vi "Begin.vi"(8 "error in":errorcluster) -> (0 "error out":errorcluster)   [LabVIEW 2020]
doc: "Called before other user functions, this VI is expected to open initial I/O refnums, load in file data, and do all program initialization. Notice that the <B>error out</B> terminal is simply used for data flow. Wiring it to other structures or subVIs ensures that this VI runs first."
uses:
  <vilib>/Rock Robotics/WPI/SafetyOutput/WPI_SafetyOutputConfigMenu.ctl
  <vilib>/Rock Robotics/WPI/DriverStation/WPI_DriverStationRobotMode2.ctl
  <vilib>/Rock Robotics/WPI/Joystick/WPI_JoystickDeviceEnum.ctl
  <vilib>/Rock Robotics/WPI/ThirdParty/REV Robotics/REVLib/Typedef/Spark MAX Motor Type.ctl
  <vilib>/Rock Robotics/SystemInterfaces/DIO/FPGA_DIOChannel.ctl
  <vilib>/Rock Robotics/SystemInterfaces/AI/FPGA_AIChannel.ctl
  <vilib>/Rock Robotics/WPI/ThirdParty/REV Robotics/REVLib/Typedef/Spark MAX Sensor Type.ctl
  Robot Global Data.vi
  <vilib>/Rock Robotics/Network Tables/NT Write String Array.vi
  <vilib>/Rock Robotics/WPI/RobotDrive/WPI_RobotDriveOpen2MotorWithExistingMotors.vi
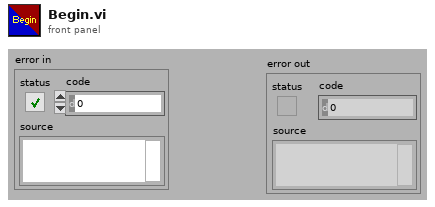
[diagram p1: front panel]
types:
  T1 = typedef "Spark MAX Sensor Type.ctl" = enum16{"No Sensor", "Hall Sensor", "Encoder", "-Not Available-", "Analog", "Alternate Encoder", "Duty Cycle"}
  T2 = typedef "FPGA_AIChannel.ctl" = enum8{"AI 0", "AI 1", "AI 2", "AI 3", "AI MXP 0", "AI MXP 1", "AI MXP 2", "AI MXP 3", "Invalid"}
  T3 = typedef "FPGA_DIOChannel.ctl" = enum8{"DIO 0", "DIO 1", "DIO 2", "DIO 3", "DIO 4", "DIO 5", "DIO 6", "DIO 7", "DIO 8", "DIO 9", "DIO MXP 0", "DIO MXP 1", "DIO MXP 2", "DIO MXP 3", "DIO MXP 4", "DIO MXP 5", "DIO MXP 6", "DIO MXP 7", "DIO MXP 8", "DIO MXP 9", "DIO MXP 10", "DIO MXP 11", "DIO MXP 12", "DIO MXP 13", "DIO MXP 14", "DIO MXP 15", "SPI Port CS1", "SPI Port CS2", "SPI Port CS3", "SPI Port MISO", "SPI Port MOSI", "Invalid"}
  T4 = typedef "Spark MAX Motor Type.ctl" = enum16{"Brushed", "Brushless"}
  T5 = typedef "WPI_JoystickDeviceEnum.ctl" = enum16{"USB 0", "USB 1", "USB 2", "USB 3", "USB 4", "USB 5"}
  T6 = typedef "WPI_DriverStationRobotMode2.ctl" = enum16{"Autonomous Disabled", "Autonomous Enabled", "Teleop Disabled", "Teleop Enabled", "Disconnected", "Finish", "Test Disabled", "Test Enabled", "Emergency Stopped"}
  T7 = typedef "WPI_SafetyOutputConfigMenu.ctl" = enum16{"Enable", "Disable"}
  T8 = typedef "WPI_MotorControlDeviceRef.ctl" = cluster{"DeviceStatus":errorcluster, "Type":T9, "PWM":cluster{"PWM Channel":T10, "DeadBand":T11}, "CAN":cluster{"Device Number":u8, "SetOutput VI Ref":variant, "GetOutput VI Ref":variant, "Enable VI Ref":variant, "Disable VI Ref":variant, "Data":variant}, "Invert":bool, "DIO PWM":cluster{"PWM \"Enable\" Channel":T10, "DIOChannel":T3, "PWM Rate":dbl}}
  T9 = typedef "WPI_MotorControlType.ctl" = enum16{"PWM", "CAN", "DIO PWM"}
  T10 = typedef "FPGA_DIOPWMChannel.ctl" = enum8{"PWM 0", "PWM 1", "PWM 2", "PWM 3", "PWM 4", "PWM 5", "PWM 6", "PWM 7", "PWM 8", "PWM 9", "PWM MXP 0", "PWM MXP 1", "PWM MXP 2", "PWM MXP 3", "PWM MXP 4", "PWM MXP 5", "PWM MXP 6", "PWM MXP 7", "PWM MXP 8", "PWM MXP 9", "Invalid"}
  T11 = typedef "WPI_PWMDeadband.ctl" = cluster{"Name":string, "maxPositivePwm":i32, "minPositivePwm":i32, "centerPwm":i32, "maxNegativePwm":i32, "minNegativePwm":i32, "angularRange":u16}
  T12 = typedef "WPI_RobotDriveDevRef.ctl" = cluster{"DevStatus":errorcluster, "Motors[]":T8[], "Square Inputs":bool, "Max Output":dbl}
  T13 = typedef "WPI_JoystickDevRef.ctl" = cluster{"Device":T5}
  T14 = typedef "WPI_DigitalOutputDevRef.ctl" = cluster{"DIO Channel":T3, "DevStatus":errorcluster}
  T15 = typedef "WPI_AnalogChannelDevRef.ctl" = cluster{"DevStatus":errorcluster, "Analog Channel":T2}
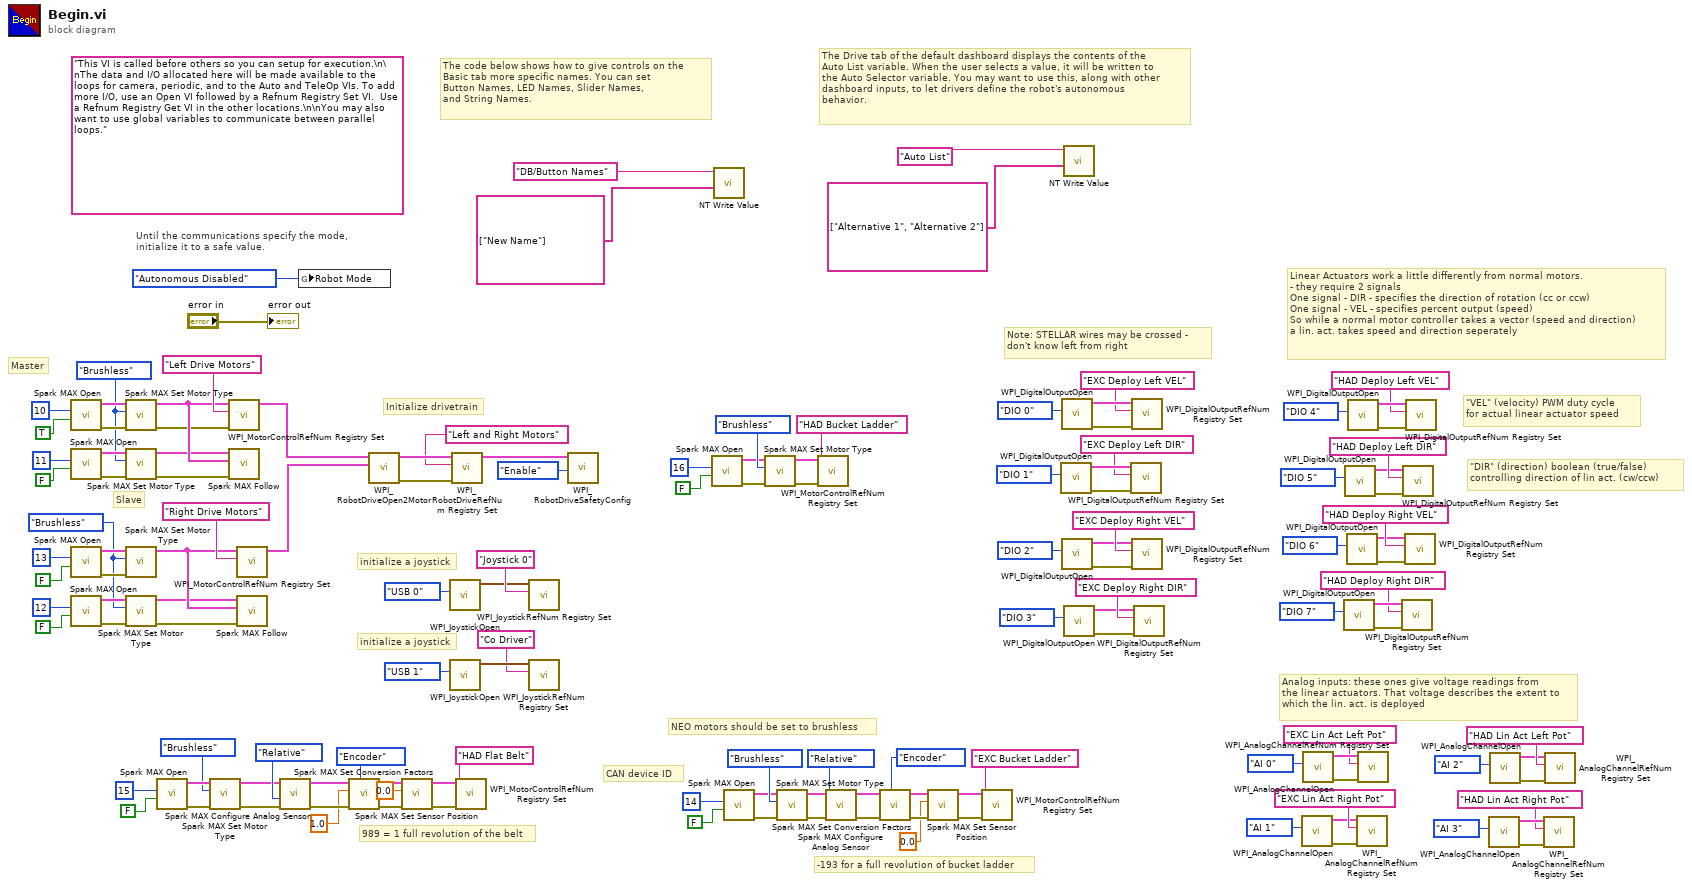
[diagram p0: block diagram]
diagram:
  w99 = Spark_MAX_Motor_Type."Brushless" ("Motor Type")
  w100 = Spark_MAX_Motor_Type."Brushless" ("Motor Type")
  (unwired) "This VI is called before others so you can setup for execution.\n\nThe data and I/O allocated here will be made available to the loops for camera, periodic, and to the Auto and TeleOp VIs. To add more I/O, use an Open VI followed by a Refnum Registry Set VI.  Use a Refnum Registry Get VI in the other locations.\n\nYou may also want to use global variables to communicate between parallel loops."
  # "-193 for a full revolution of bucket ladder"
  # "989 = 1 full revolution of the belt"
  # "Initialize drivetrain"
  # "Analog inputs: these ones give voltage readings from\nthe linear actuators. That voltage describes the extent to\nwhich the lin. act. is deployed"
  # "Slave"
  # "Master"
  # "CAN device ID"
  # "Linear Actuators work a little differently from normal motors.\n- they require 2 signals\nOne signal - DIR - specifies the direction of rotation (cc or ccw)\nOne signal - VEL - specifies percent output (speed)\nSo while a normal motor controller takes a vector (speed and direction)\na lin. act. takes speed and direction seperately"
  # "\"DIR\" (direction) boolean (true/false)\ncontrolling direction of lin act. (cw/ccw)"
  # "\"VEL\" (velocity) PWM duty cycle \nfor actual linear actuator speed"
  # "NEO motors should be set to brushless"
  # "Note: STELLAR wires may be crossed - \ndon't know left from right"
  # "initialize a joystick"
  # "The Drive tab of the default dashboard displays the contents of the\nAuto List variable. When the user selects a value, it will be written to\nthe Auto Selector variable. You may want to use this, along with other\ndashboard inputs, to let drivers define the robot's autonomous\nbehavior."
  # "The code below shows how to give controls on the\nBasic tab more specific names. You can set\nButton Names, LED Names, Slider Names,\nand String Names."
  # "initialize a joystick"
  # "Until the communications specify the mode,\ninitialize it to a safe value."
  n1 = call <vilib>:"Spark MAX Open.vi"("Invert"=TRUE, "Device Number"=u8 10) -> ("error out"=w107:errorcluster, "MotorControlDeviceRef"=w108:T8)  [unwired: 8 in]
  n2 = call <vilib>:"Spark MAX Open.vi"("Invert"=FALSE, "Device Number"=u8 11) -> ("error out"=w106:errorcluster, "MotorControlDeviceRef"=w105:T8)  [unwired: 8 in]
  n3 = call <vilib>:"Spark MAX Open.vi"("Invert"=FALSE, "Device Number"=u8 13) -> ("error out"=w104:errorcluster, "MotorControlDeviceRef"=w103:T8)  [unwired: 8 in]
  n4 = call <vilib>:"Spark MAX Open.vi"("Invert"=FALSE, "Device Number"=u8 12) -> ("error out"=w102:errorcluster, "MotorControlDeviceRef"=w101:T8)  [unwired: 8 in]
  n5 = call <vilib>:"Spark MAX Set Motor Type.vi"("error in (no error)"=w107, "Motor Type"=w100, "MotorControlDevRef"=w108) -> ("error out"=w45:errorcluster, "MotorControlDeviceRef"=w46:T8)  [unwired: 7 in]
  n6 = call <vilib>:"Spark MAX Set Motor Type.vi"("error in (no error)"=w106, "Motor Type"=w100, "MotorControlDevRef"=w105) -> ("error out"=w44:errorcluster, "MotorControlDeviceRef"=w43:T8)  [unwired: 7 in]
  n7 = call <vilib>:"Spark MAX Set Motor Type.vi"("error in (no error)"=w104, "Motor Type"=w99, "MotorControlDevRef"=w103) -> ("MotorControlDeviceRef"=w42:T8)  [unwired: 7 in, 1 out]
  n8 = call <vilib>:"Spark MAX Set Motor Type.vi"("error in (no error)"=w102, "Motor Type"=w99, "MotorControlDevRef"=w101) -> ("error out"=w41:errorcluster, "MotorControlDeviceRef"=w40:T8)  [unwired: 7 in]
  n9 = call <vilib>:"Spark MAX Open.vi"("Invert"=FALSE, "Device Number"=u8 15) -> ("error out"=w92:errorcluster, "MotorControlDeviceRef"=w91:T8)  [unwired: 8 in]
  n10 = call <vilib>:"Spark MAX Set Motor Type.vi"("error in (no error)"=w92, "Motor Type"=Spark_MAX_Motor_Type."Brushless", "MotorControlDevRef"=w91) -> ("error out"=w21:errorcluster, "MotorControlDeviceRef"=w22:T8)  [unwired: 7 in]
  n11 = call <vilib>:"WPI_MotorControlRefNum Registry Set.vi"("error in (no error)"=w45, "refnum name"="Left Drive Motors", "MotorControlDevRef"=w46) -> ("MotorControlDevRef"=w110:T8)  [unwired: 7 in, 1 out]
  n12 = call <vilib>:"Spark MAX Follow.vi"("error in (no error)"=w44, "Master Controller"=w46, "MotorControlDeviceRef"=w43) -> ()  [unwired: 7 in, 2 out]
  n13 = call <vilib>:"WPI_MotorControlRefNum Registry Set.vi"("refnum name"="Right Drive Motors", "MotorControlDevRef"=w42) -> ("MotorControlDevRef"=w109:T8)  [unwired: 8 in, 1 out]
  n14 = call <vilib>:"Spark MAX Follow.vi"("error in (no error)"=w41, "Master Controller"=w42, "MotorControlDeviceRef"=w40) -> ()  [unwired: 7 in, 2 out]
  n15 = call <vilib>:"Spark MAX Configure Analog Sensor.vi"("error in (no error)"=w21, "Sensor Mode (Absolute)"=enum16{"Absolute", "Relative"}."Relative", "MotorControlDeviceRef in"=w22) -> ("error out"=w19:errorcluster, "MotorControlDeviceRef"=w20:T8)  [unwired: 7 in]
  n16 = global write "Robot Global Data.vi" "Robot Mode"(WPI_DriverStationRobotMode2."Autonomous Disabled" ("Robot Mode")) -> ()
  n17 = call <vilib>:"Spark MAX Set Conversion Factors.vi"("Sensor Type (Hall Sensor)"=Spark_MAX_Sensor_Type."Encoder", "error in (no error)"=w19, "Position Factor (1)"=1.0, "MotorControlDeviceRef in"=w20) -> ("error out"=w16:errorcluster, "MotorControlDeviceRef out"=w15:T8)  [unwired: 6 in]
  n18 = call-poly <vilib>:"WPI_RobotDriveOpen2Motor.vi"("Right Motor Dev Ref"=w109, "Left Motor Dev Ref"=w110) -> ("error out"=w135:errorcluster, "RobotDriveDevRef"=w137:T12)  [unwired: 3 in, 5 out]
  n19 = call <vilib>:"Spark MAX Set Sensor Position.vi"("error in"=w16, "Position"=0.0, "MotorControlDeviceRef"=w15) -> ("error out"=w13:errorcluster, "MotorControlDeviceRef"=w14:T8)  [unwired: 7 in]
  n20 = call <vilib>:"WPI_JoystickOpen.vi"("JoystickDevice"=WPI_JoystickDeviceEnum."USB 0") -> ("JoystickDevRef"=w130:T13)  [unwired: 10 in]
  n21 = call <vilib>:"WPI_JoystickOpen.vi"("JoystickDevice"=WPI_JoystickDeviceEnum."USB 1") -> ("JoystickDevRef"=w122:T13)  [unwired: 10 in]
  n22 = call <vilib>:"WPI_RobotDriveRefNum Registry Set.vi"("error in (no error)"=w135, "refnum name"="Left and Right Motors", "RobotDriveDevRef"=w137) -> ("RobotDriveDevRef"=w134:T12)  [unwired: 1 in, 7 out]
  n23 = call <vilib>:"WPI_MotorControlRefNum Registry Set.vi"("error in (no error)"=w13, "refnum name"="HAD Flat Belt", "MotorControlDevRef"=w14) -> ()  [unwired: 7 in, 2 out]
  n24 = call <vilib>:"WPI_JoystickRefNum Registry Set.vi"("refnum name"="Joystick 0", "JoystickDevRef"=w130) -> ()  [unwired: 8 in, 2 out]
  n25 = call <vilib>:"WPI_JoystickRefNum Registry Set.vi"("refnum name"="Co Driver", "JoystickDevRef"=w122) -> ()  [unwired: 8 in, 2 out]
  n26 = call <vilib>:"WPI_RobotDriveSafetyConfig.vi"("mode"=WPI_SafetyOutputConfigMenu."Enable", "RobotDriveDevRef"=w134) -> ()  [unwired: 8 in, 2 out]
  n27 = call <vilib>:"Spark MAX Open.vi"("Invert"=FALSE, "Device Number"=u8 16) -> ("error out"=w79:errorcluster, "MotorControlDeviceRef"=w80:T8)  [unwired: 8 in]
  n28 = call-poly <vilib>:"NT Write Value.vi"("value"=string[] ["New Name"], "name"="DB/Button Names" ("Name")) -> ()  [unwired: 9 in, 1 out]
  n29 = call <vilib>:"Spark MAX Open.vi"("Invert"=FALSE, "Device Number"=u8 14) -> ("error out"=w93:errorcluster, "MotorControlDeviceRef"=w94:T8)  [unwired: 8 in]
  n30 = call <vilib>:"Spark MAX Set Motor Type.vi"("error in (no error)"=w79, "Motor Type"=Spark_MAX_Motor_Type."Brushless", "MotorControlDevRef"=w80) -> ("error out"=w81:errorcluster, "MotorControlDeviceRef"=w82:T8)  [unwired: 7 in]
  n31 = call <vilib>:"Spark MAX Set Motor Type.vi"("error in (no error)"=w93, "Motor Type"=Spark_MAX_Motor_Type."Brushless", "MotorControlDevRef"=w94) -> ("error out"=w11:errorcluster, "MotorControlDeviceRef"=w10:T8)  [unwired: 7 in]
  n32 = call <vilib>:"WPI_MotorControlRefNum Registry Set.vi"("error in (no error)"=w81, "refnum name"="HAD Bucket Ladder", "MotorControlDevRef"=w82) -> ()  [unwired: 7 in, 2 out]
  n33 = call <vilib>:"Spark MAX Configure Analog Sensor.vi"("error in (no error)"=w11, "Sensor Mode (Absolute)"=enum16{"Absolute", "Relative"}."Relative", "MotorControlDeviceRef in"=w10) -> ("error out"=w8:errorcluster, "MotorControlDeviceRef"=w9:T8)  [unwired: 7 in]
  n34 = call <vilib>:"Spark MAX Set Conversion Factors.vi"("Sensor Type (Hall Sensor)"=Spark_MAX_Sensor_Type."Encoder", "error in (no error)"=w8, "MotorControlDeviceRef in"=w9) -> ("error out"=w7:errorcluster, "MotorControlDeviceRef out"=w6:T8)  [unwired: 7 in]
  n35 = call <vilib>:"Spark MAX Set Sensor Position.vi"("error in"=w7, "Position"=0.0, "MotorControlDeviceRef"=w6) -> ("error out"=w4:errorcluster, "MotorControlDeviceRef"=w5:T8)  [unwired: 7 in]
  n36 = call <vilib>:"WPI_MotorControlRefNum Registry Set.vi"("error in (no error)"=w4, "refnum name"="EXC Bucket Ladder", "MotorControlDevRef"=w5) -> ()  [unwired: 7 in, 2 out]
  n37 = call <vilib>:"WPI_DigitalOutputOpen.vi"("DIO Channel"=FPGA_DIOChannel."DIO 1") -> ("error out"=w78:errorcluster, "DigitalOutputDevRef"=w77:T14)  [unwired: 9 in]
  n38 = call <vilib>:"WPI_DigitalOutputOpen.vi"("DIO Channel"=FPGA_DIOChannel."DIO 0") -> ("error out"=w74:errorcluster, "DigitalOutputDevRef"=w73:T14)  [unwired: 9 in]
  n39 = call <vilib>:"WPI_DigitalOutputOpen.vi"("DIO Channel"=FPGA_DIOChannel."DIO 2") -> ("error out"=w67:errorcluster, "DigitalOutputDevRef"=w68:T14)  [unwired: 9 in]
  n40 = call-poly <vilib>:"NT Write Value.vi"("value"=string[] ["Alternative 1", "Alternative 2"] ("String Array"), "name"="Auto List" ("Name")) -> ()  [unwired: 9 in, 1 out]
  n41 = call <vilib>:"WPI_DigitalOutputOpen.vi"("DIO Channel"=FPGA_DIOChannel."DIO 3") -> ("error out"=w63:errorcluster, "DigitalOutputDevRef"=w64:T14)  [unwired: 9 in]
  n42 = call <vilib>:"WPI_DigitalOutputRefNum Registry Set.vi"("error in (no error)"=w78, "refnum name"="EXC Deploy Left DIR", "DigitalOutputDevRef"=w77) -> ()  [unwired: 7 in, 2 out]
  n43 = call <vilib>:"WPI_DigitalOutputRefNum Registry Set.vi"("error in (no error)"=w74, "refnum name"="EXC Deploy Left VEL", "DigitalOutputDevRef"=w73) -> ()  [unwired: 7 in, 2 out]
  n44 = call <vilib>:"WPI_DigitalOutputRefNum Registry Set.vi"("error in (no error)"=w67, "refnum name"="EXC Deploy Right VEL", "DigitalOutputDevRef"=w68) -> ()  [unwired: 7 in, 2 out]
  n45 = call <vilib>:"WPI_DigitalOutputRefNum Registry Set.vi"("error in (no error)"=w63, "refnum name"="EXC Deploy Right DIR", "DigitalOutputDevRef"=w64) -> ()  [unwired: 7 in, 2 out]
  n46 = call <vilib>:"WPI_AnalogChannelOpen.vi"("Analog Channel"=FPGA_AIChannel."AI 1") -> ("error out"=w32:errorcluster, "AIDeviceRef"=w33:T15)  [unwired: 9 in]
  n47 = call <vilib>:"WPI_AnalogChannelOpen.vi"("Analog Channel"=FPGA_AIChannel."AI 0") -> ("error out"=w39:errorcluster, "AIDeviceRef"=w38:T15)  [unwired: 9 in]
  n48 = call <vilib>:"WPI_DigitalOutputOpen.vi"("DIO Channel"=FPGA_DIOChannel."DIO 7") -> ("error out"=w54:errorcluster, "DigitalOutputDevRef"=w53:T14)  [unwired: 9 in]
  n49 = call <vilib>:"WPI_DigitalOutputOpen.vi"("DIO Channel"=FPGA_DIOChannel."DIO 5") -> ("error out"=w55:errorcluster, "DigitalOutputDevRef"=w56:T14)  [unwired: 9 in]
  n50 = call <vilib>:"WPI_DigitalOutputOpen.vi"("DIO Channel"=FPGA_DIOChannel."DIO 6") -> ("error out"=w47:errorcluster, "DigitalOutputDevRef"=w48:T14)  [unwired: 9 in]
  n51 = call <vilib>:"WPI_DigitalOutputOpen.vi"("DIO Channel"=FPGA_DIOChannel."DIO 4") -> ("error out"=w62:errorcluster, "DigitalOutputDevRef"=w61:T14)  [unwired: 9 in]
  n52 = call <vilib>:"WPI_AnalogChannelRefNum Registry Set.vi"("error in (no error)"=w32, "refnum name"="EXC Lin Act Right Pot", "AIDeviceRef"=w33) -> ()  [unwired: 7 in, 2 out]
  n53 = call <vilib>:"WPI_AnalogChannelRefNum Registry Set.vi"("error in (no error)"=w39, "refnum name"="EXC Lin Act Left Pot", "AIDeviceRef"=w38) -> ()  [unwired: 7 in, 2 out]
  n54 = call <vilib>:"WPI_DigitalOutputRefNum Registry Set.vi"("error in (no error)"=w54, "refnum name"="HAD Deploy Right DIR", "DigitalOutputDevRef"=w53) -> ()  [unwired: 7 in, 2 out]
  n55 = call <vilib>:"WPI_DigitalOutputRefNum Registry Set.vi"("error in (no error)"=w55, "refnum name"="HAD Deploy Left DIR", "DigitalOutputDevRef"=w56) -> ()  [unwired: 7 in, 2 out]
  n56 = call <vilib>:"WPI_DigitalOutputRefNum Registry Set.vi"("error in (no error)"=w47, "refnum name"="HAD Deploy Right VEL", "DigitalOutputDevRef"=w48) -> ()  [unwired: 7 in, 2 out]
  n57 = call <vilib>:"WPI_DigitalOutputRefNum Registry Set.vi"("error in (no error)"=w62, "refnum name"="HAD Deploy Left VEL", "DigitalOutputDevRef"=w61) -> ()  [unwired: 7 in, 2 out]
  n58 = call <vilib>:"WPI_AnalogChannelOpen.vi"("Analog Channel"=FPGA_AIChannel."AI 3") -> ("error out"=w31:errorcluster, "AIDeviceRef"=w30:T15)  [unwired: 9 in]
  n59 = call <vilib>:"WPI_AnalogChannelOpen.vi"("Analog Channel"=FPGA_AIChannel."AI 2") -> ("error out"=w24:errorcluster, "AIDeviceRef"=w25:T15)  [unwired: 9 in]
  n60 = call <vilib>:"WPI_AnalogChannelRefNum Registry Set.vi"("error in (no error)"=w31, "refnum name"="HAD Lin Act Right Pot", "AIDeviceRef"=w30) -> ()  [unwired: 7 in, 2 out]
  n61 = call <vilib>:"WPI_AnalogChannelRefNum Registry Set.vi"("error in (no error)"=w24, "refnum name"="HAD Lin Act Left Pot", "AIDeviceRef"=w25) -> ()  [unwired: 7 in, 2 out]
  "error out" <- "error in"
